vi "GenChnl2CleanTask.vi"(11 "Generated Channel In":string) -> (2 "Channel Out":string)   [LabVIEW 2013]
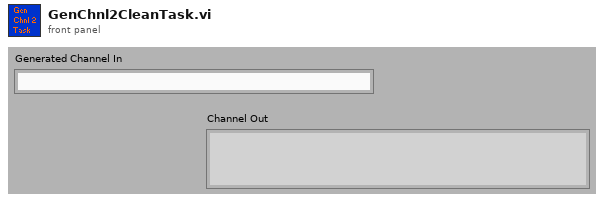
[diagram p1: front panel]
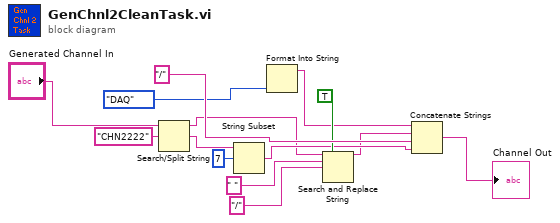
[diagram p0: block diagram]
diagram:
  n1 = Search/Split String(string="Generated Channel In", search string/char (-)="CHN2222") -> (substring before match=w4:string, match + rest of string=w12:string)  [unwired: 2 out]
  n2 = String Subset(string=w12, offset (0)=7) -> (substring=w5:string)  [unwired: 1 out]
  n3 = Format Into String(enum16{"DAQ", "Operations Manager", "Generated"}."DAQ" ("Source")) -> (resulting string=w1:string)  [unwired: 3 in, 1 out]
  n4 = Search and Replace String(replace all?=TRUE ("replace all? (F)"), input string=w4, search string=" ", replace string="/" ("replace string (\"\")")) -> (result string=w3:string)  [unwired: 1 in, 6 out]
  n5 = Concatenate Strings(w1, w3, "/" ("string"), w5) -> (→"Channel Out":string)
